vi "RSZVB Get Group Of All Measured Ports.vi"(8 "error in (no error)":errorcluster {"code" format="%.0x"}, 9 "Group (1)":i32=1, 10 "Channel (1)":i32=1, 11 "VISA session":refnum<visa-resource-name>) -> (0 "error out":errorcluster {"code" format="%.0x"}, 3 "dup VISA session":refnum<visa-resource-name>, 5 "Ports":i32[](array[numeric]))   [LabVIEW 2011]
doc: "This VI returns a port group numbered <group_no> containing an arbitrary selection of logical ports.\n\nRemote-control command(s):\nSOURce<Ch>:GROup<group_no>:PORTs?"
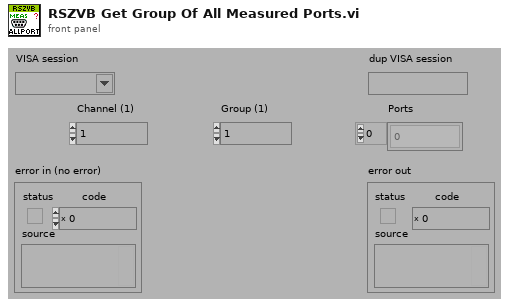
[diagram p1: front panel]
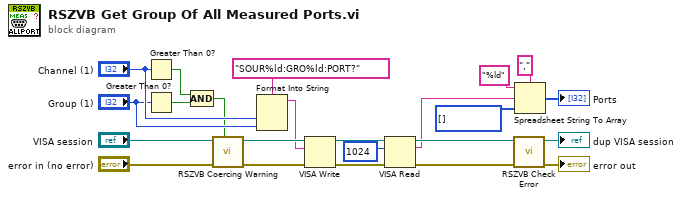
[diagram p0: block diagram]
diagram:
  n1 = Greater Than 0?(x="Channel (1)") -> (x > 0?=w15:bool)
  n2 = Greater Than 0?(x="Group (1)") -> (x > 0?=w16:bool)
  n3 = Compound Arithmetic op=AND(w15, w16) -> (w18:bool)
  n4 = call "RSZVB Coercing Warning.vi"("In Range?"=w18, "error in (no error)"="error in (no error)", "VISA session"="VISA session") -> ("error out"=w19:errorcluster, "dup VISA session"=w20:refnum<visa-resource-name>)  [unwired: 7 in]
  n5 = Format Into String(format string="SOUR%ld:GRO%ld:PORT?", "Channel (1)", "Group (1)") -> (resulting string=w17:string)  [unwired: 2 in, 1 out]
  n6 = VISA Write(VISA resource name=w20, write buffer=w17, error in (no error)=w19) -> (VISA resource name out=w10:refnum<visa-resource-name>, error out=w9:errorcluster)  [unwired: 1 out]
  n7 = VISA Read(VISA resource name=w10, byte count=u32 1024 ("byte count (0)"), error in (no error)=w9) -> (VISA resource name out=w7:refnum<visa-resource-name>, read buffer=w1:string, error out=w6:errorcluster)  [unwired: 1 out]
  n8 = call "RSZVB Check Error.vi"("error in (no error)"=w6, "VISA session"=w7) -> ("error out"=→"error out":errorcluster, "dup VISA session"=→"dup VISA session":refnum<visa-resource-name>)  [unwired: 8 in]
  n9 = Spreadsheet String To Array(delimiter (Tab)=",", format string="%ld", spreadsheet string=w1, array type (2D Dbl)=i32[] []) -> (array=→"Ports":i32[])
